vi "PTRead.vi"(0 "Array in":dbl[](array[numeric]), 1 "P06":dbl, 2 "P03":dbl, 3 "P06 1":dbl, 4 "P03 1":dbl, 5 "P07":dbl, 6 "P04":dbl, 7 "P07 1":dbl, 8 "P01":dbl, 9 "P08":dbl, 10 "P01 1":dbl, 11 "P04 1":dbl, 12 "P02":dbl, 13 "P08 1":dbl, 14 "P02 1":dbl, 15 "P09":dbl, 16 "P05":dbl, 17 "P09 1":dbl, 18 "P05 1":dbl, 19 "atm":dbl) -> (20 "Array out":dbl[](array[numeric]))   [LabVIEW 2017]
doc: "Reads the current input from the pressure transducers"
panel:
  out "AI6":dbl
  out "AI0":dbl
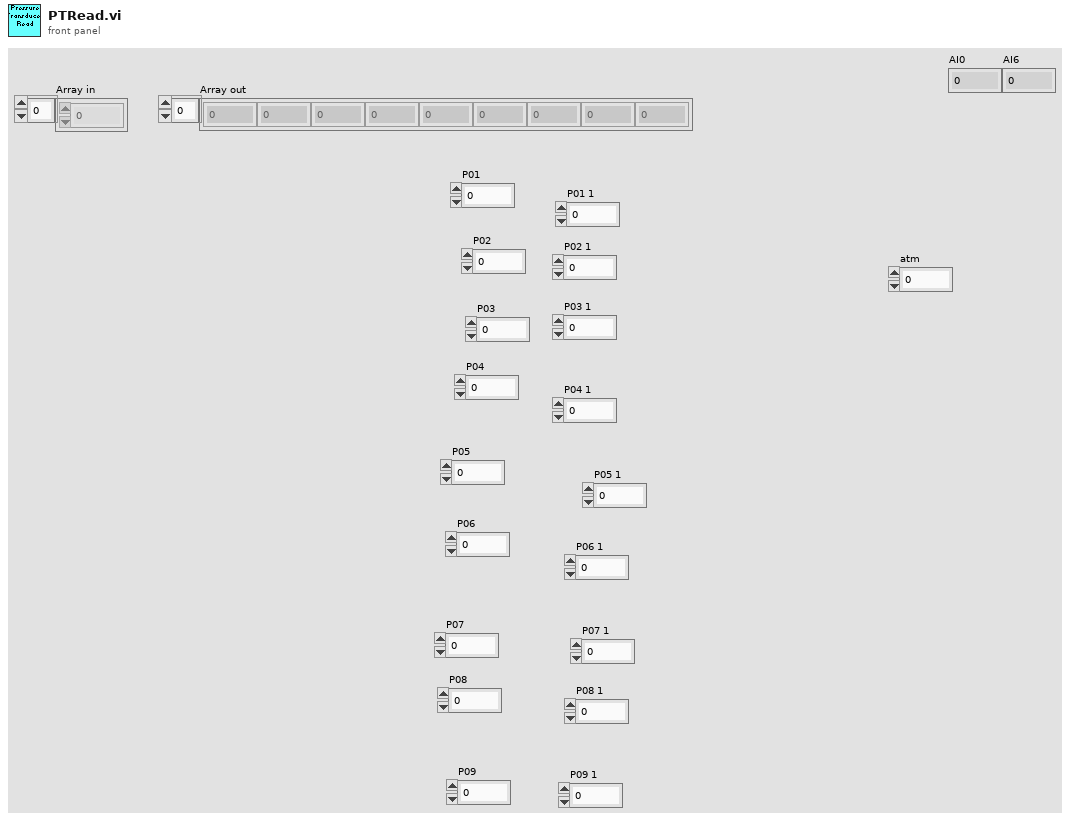
[diagram p1: front panel]
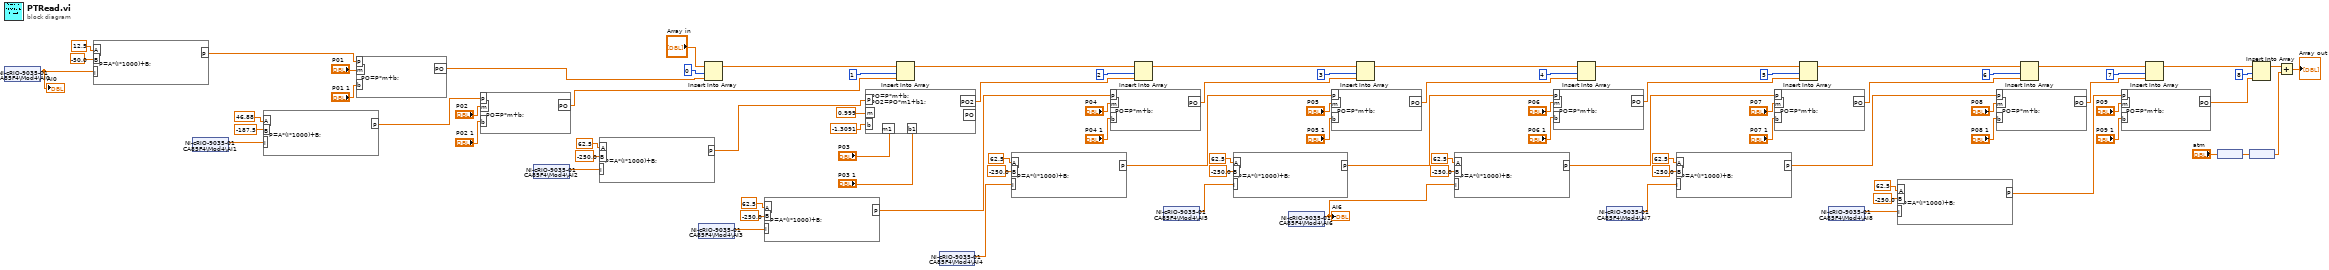
[diagram p0: block diagram]
diagram:
  n1 = shared-variable "NI-cRIO-9035-01CA85F4\\Mod4\\AI0"() -> (w53:dbl)  [unwired: 1 in, 1 out]
  "AI0" <- w53
  n2 = formula code="P=A*(I*1000)+B;"("I"=w53, "A"=12.5 ("input variable"), "B"=-50.0 ("input variable")) -> ("P"=w33:dbl)
  n3 = shared-variable "NI-cRIO-9035-01CA85F4\\Mod4\\AI1"() -> (w57:dbl)  [unwired: 1 in, 1 out]
  n4 = formula code="P=A*(I*1000)+B;"("I"=w57, "A"=46.88 ("input variable"), "B"=-187.5 ("input variable")) -> ("P"=w30:dbl)
  n5 = formula code="PO=P*m+b;"("m"="P01", "b"="P01 1", "P"=w33) -> ("PO"=w2:dbl)
  n6 = formula code="PO=P*m+b;"("m"="P02", "b"="P02 1", "P"=w30) -> ("PO"=w1:dbl)
  n7 = shared-variable "NI-cRIO-9035-01CA85F4\\Mod4\\AI2"() -> (w63:dbl)  [unwired: 1 in, 1 out]
  n8 = formula code="P=A*(I*1000)+B;"("I"=w63, "A"=62.5 ("input variable"), "B"=-250.0 ("input variable")) -> ("P"=w41:dbl)
  n9 = shared-variable "NI-cRIO-9035-01CA85F4\\Mod4\\AI3"() -> (w66:dbl)  [unwired: 1 in, 1 out]
  n10 = Insert Into Array(array="Array in", index=0, new element=w2) -> (w60:dbl[])
  n11 = formula code="P=A*(I*1000)+B;"("I"=w66, "A"=62.5 ("input variable"), "B"=-250.0 ("input variable")) -> ("P"=w35:dbl)
  n12 = formula code="PO=P*m+b;\nPO2=PO*m1+b1;"("P"=w41, "m"=0.999 ("Numeric"), "b"=-1.3091 ("Numeric 2"), "m1"="P03", "b1"="P03 1") -> ("PO2"=w38:dbl)  [unwired: 1 out]
  n13 = Insert Into Array(array=w60, index=1, new element=w1) -> (w82:dbl[])
  n14 = shared-variable "NI-cRIO-9035-01CA85F4\\Mod4\\AI4"() -> (w69:dbl)  [unwired: 1 in, 1 out]
  n15 = formula code="P=A*(I*1000)+B;"("I"=w69, "A"=62.5 ("input variable"), "B"=-250.0 ("input variable")) -> ("P"=w27:dbl)
  n16 = formula code="PO=P*m+b;"("m"="P04", "b"="P04 1", "P"=w35) -> ("PO"=w34:dbl)
  n17 = Insert Into Array(array=w82, index=2, new element=w38) -> (w83:dbl[])
  n18 = shared-variable "NI-cRIO-9035-01CA85F4\\Mod4\\AI5"() -> (w72:dbl)  [unwired: 1 in, 1 out]
  n19 = formula code="P=A*(I*1000)+B;"("I"=w72, "A"=62.5 ("input variable"), "B"=-250.0 ("input variable")) -> ("P"=w23:dbl)
  n20 = shared-variable "NI-cRIO-9035-01CA85F4\\Mod4\\AI6"() -> (w75:dbl)  [unwired: 1 in, 1 out]
  "AI6" <- w75
  n21 = formula code="PO=P*m+b;"("m"="P05", "b"="P05 1", "P"=w27) -> ("PO"=w24:dbl)
  n22 = Insert Into Array(array=w83, index=3, new element=w34) -> (w84:dbl[])
  n23 = formula code="P=A*(I*1000)+B;"("I"=w75, "A"=62.5 ("input variable"), "B"=-250.0 ("input variable")) -> ("P"=w19:dbl)
  n24 = formula code="PO=P*m+b;"("m"="P06", "b"="P06 1", "P"=w23) -> ("PO"=w20:dbl)
  n25 = Insert Into Array(array=w84, index=4, new element=w24) -> (w85:dbl[])
  n26 = shared-variable "NI-cRIO-9035-01CA85F4\\Mod4\\AI7"() -> (w80:dbl)  [unwired: 1 in, 1 out]
  n27 = formula code="P=A*(I*1000)+B;"("I"=w80, "A"=62.5 ("input variable"), "B"=-250.0 ("input variable")) -> ("P"=w15:dbl)
  n28 = formula code="PO=P*m+b;"("m"="P07", "b"="P07 1", "P"=w19) -> ("PO"=w16:dbl)
  n29 = Insert Into Array(array=w85, index=5, new element=w20) -> (w86:dbl[])
  n30 = shared-variable "NI-cRIO-9035-01CA85F4\\Mod4\\AI8"() -> (w81:dbl)  [unwired: 1 in, 1 out]
  n31 = formula code="P=A*(I*1000)+B;"("I"=w81, "A"=62.5 ("input variable"), "B"=-250.0 ("input variable")) -> ("P"=w11:dbl)
  n32 = formula code="PO=P*m+b;"("m"="P08", "b"="P08 1", "P"=w15) -> ("PO"=w12:dbl)
  n33 = Insert Into Array(array=w86, index=6, new element=w16) -> (w87:dbl[])
  n34 = formula code="PO=P*m+b;"("m"="P09", "b"="P09 1", "P"=w11) -> ("PO"=w8:dbl)
  n35 = Insert Into Array(array=w87, index=7, new element=w12) -> (w88:dbl[])
  n36 = node("atm") -> (w6:dbl[unit])
  n37 = node(w6) -> (w3:dbl)
  n38 = Insert Into Array(array=w88, index=8, new element=w8) -> (w5:dbl[])
  n39 = Add(x=w5, y=w3) -> (x+y=→"Array out":dbl[])
